vi "Initialize.vi"(8 "error in (no error)":errorcluster, 9 "Reset? (T: Yes)":bool=TRUE, 10 "ID Query? (T: Yes)":bool=TRUE, 11 "VISA resource name":refnum<visa-resource-name>) -> (0 "error out":errorcluster, 3 "VISA resource name out":refnum<visa-resource-name>)   [LabVIEW 2017, in "Agilent 6000 Series.lvlib"]
doc: "Establishes communication with the instrument and optionally performs an instrument identification query and/or an instrument reset. It also places the instrument in a default state needed for other instrument driver operations. Therefore, call this VI before calling other instrument driver VIs for this instrument. Generally, you need to call the <B>Initialize VI</B> only once at the beginning of an application."
uses:
  <instrlib>/Agilent 6000 Series/Agilent 6000 Series.lvlib
  <vilib>/regexp/Match Regular Expression.xnode
panel:
  # "(c) 2009-2015 National Instruments.  ALL RIGHTS RESERVED."
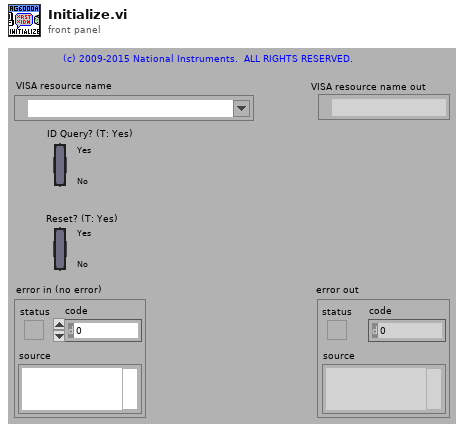
[diagram p1: front panel]
types:
  T1 = cluster{"Status":bool, "Code":i32, "Source (VI Name)":string}
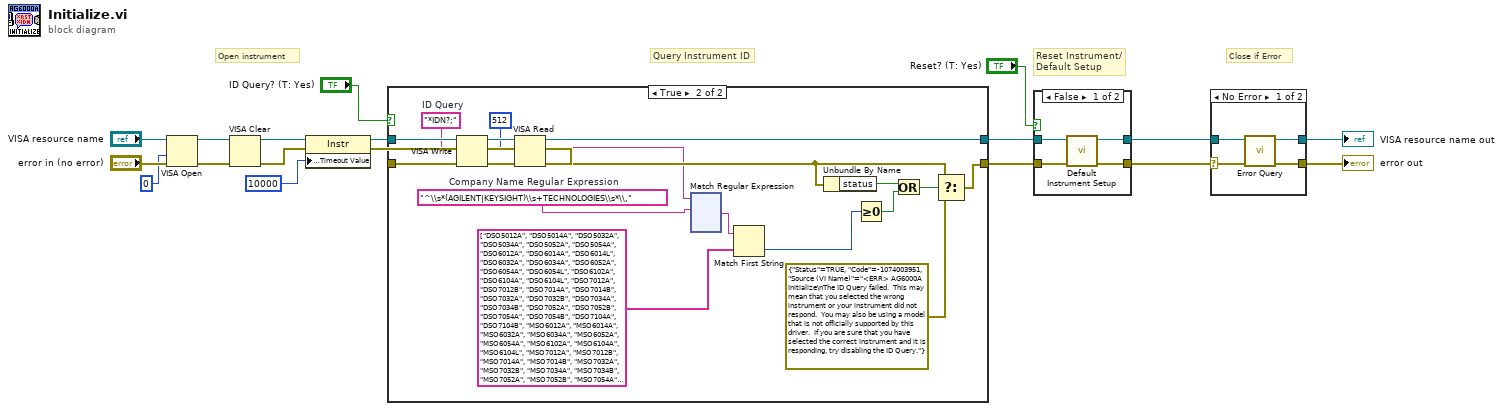
[diagram p0: block diagram]
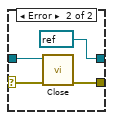
[diagram p2: hidden frame]
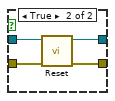
[diagram p3: hidden frame]
diagram:
  # "Close if Error"
  # "Query Instrument ID"
  # "Reset Instrument/\nDefault Setup"
  # "Open instrument"
  n1 = VISA Open(access mode=u32 0, error in (no error)="error in (no error)", VISA resource name="VISA resource name") -> (VISA resource name=w8:refnum<visa-resource-name>, error out=w7:errorcluster)  [unwired: 2 in]
  n2 = VISA Clear(VISA resource name=w8, error in (no error)=w7) -> (VISA resource name out=w6:refnum<visa-resource-name>, error out=w5:errorcluster)
  n3 = property on="Property Node" class="Instr"(reference=w6, error in=w5, "General Settings:Timeout Value"=u32 10000) -> (reference out=w11:refnum<visa-resource-name>, error out=w10:errorcluster)
  n4 = case shown="True" "ID Query? (T: Yes)" {
    tunnel: [w19 w38] -> w17
    tunnel: [w20 w35] -> w18
    tunnel: w11 -> [w20 w36]
    tunnel: w10 -> [w19 w37]
    frame False {
    }
    frame True {
      w24 = "^\\s*(AGILENT|KEYSIGHT)\\s+TECHNOLOGIES\\s*\\,"  # Company Name Regular Expression
      w26 = "*IDN?;"  # ID Query
      n5 = VISA Write(VISA resource name=w36, write buffer=w26, error in (no error)=w37) -> (VISA resource name out=w33:refnum<visa-resource-name>, error out=w31:errorcluster)  [unwired: 1 out]
      n6 = VISA Read(VISA resource name=w33, byte count=u32 512, error in (no error)=w31) -> (VISA resource name out=w35:refnum<visa-resource-name>, read buffer=w23:string, error out=w32:errorcluster)  [unwired: 1 out]
      n7 = xnode "Match Regular Expression"("input string"=w23, "regular expression"=w24) -> ("after match"=w22:string)  [unwired: 4 in, 4 out]
      n8 = Match First String(2:string[] ["DSO5012A", "DSO5014A", "DSO5032A", "DSO5034A", "DSO5052A", "DSO5054A", "DSO6012A", "DSO6014A", "DSO6014L", "DSO6032A", "DSO6034A", "DSO6052A", "DSO6054A", "DSO6054L", "DSO6102A", "DSO6104A", "DSO6104L", "DSO7012A", "DSO7012B", "DSO7014A", "DSO7014B", "DSO7032A", "DSO7032B", "DSO7034A", "DSO7034B", "DSO7052A", "DSO7052B", "DSO7054A", "DSO7054B", "DSO7104A", "DSO7104B", "MSO6012A", "MSO6014A", "MSO6032A", "MSO6034A", "MSO6052A", "MSO6054A", "MSO6102A", "MSO6104A", "MSO6104L", "MSO7012A", "MSO7012B", "MSO7014A", "MSO7014B", "MSO7032A", "MSO7032B", "MSO7034A", "MSO7034B", "MSO7052A", "MSO7052B", "MSO7054A", "MSO7054B", "MSO7104A", "MSO7104B"] ("string array"), 3:w22) -> (0:w28:i32)  [unwired: 1 out]
      n9 = Unbundle By Name(w32) -> ("status"=w29:bool)
      n10 = Greater Or Equal To 0?(x=w28) -> (x >= 0?=w34:bool)
      n11 = Or(x=w29, y=w34) -> (x .or. y?=w30:bool)
      n12 = Select(t=w32, s=w30, f=T1 {"Status"=TRUE, "Code"=-1074003951, "Source (VI Name)"="<ERR> AG6000A Initialize\nThe ID Query failed.  This may mean that you selected the wrong instrument or your instrument did not respond.  You may also be using a model that is not officially supported by this driver.  If you are sure that you have selected the correct instrument and it is responding, try disabling the ID Query."}) -> (s? t:f=w38:T1)
    }
  }
  n13 = case shown="False" "Reset? (T: Yes)" {
    tunnel: w17 -> [w155 w157]
    tunnel: [w154 w160] -> w1
    tunnel: w18 -> [w156 w158]
    tunnel: [w153 w159] -> w2
    frame False {
      n14 = call <instrlib>:"Default Instrument Setup.vi"("error in (no error)"=w155, "VISA resource name"=w156) -> ("error out"=w154:errorcluster, "VISA resource name out"=w153:refnum<visa-resource-name>)  [unwired: 8 in]
    }
    frame True {
      n15 = call <instrlib>:"Reset.vi"("error in (no error)"=w157, "VISA resource name"=w158) -> ("error out"=w160:errorcluster, "VISA resource name out"=w159:refnum<visa-resource-name>)  [unwired: 8 in]
    }
  }
  n16 = case shown="No Error" w1 {
    selector: w1 -> [w162 w166]
    tunnel: w2 -> [w161 w167]
    tunnel: [w164 refnum<visa-resource-name> refnum ("VISA resource name out")] -> w4
    tunnel: [w163 w168] -> w3
    frame No Error {
      n17 = call <instrlib>:"Error Query.vi"("error in (no error)"=w162, "VISA resource name"=w161) -> ("error out"=w163:errorcluster, "VISA resource name out"=w164:refnum<visa-resource-name>)  [unwired: 6 in, 2 out]
    }
    frame Error {
      n18 = call <instrlib>:"Close.vi"("error in (no error)"=w166, "VISA resource name"=w167) -> ("error out"=w168:errorcluster)  [unwired: 9 in]
    }
  }
  "VISA resource name out" <- w4
  "error out" <- w3
